vi "未命名 5.vi"() -> ()   [LabVIEW 2012, in "DataGridView.lvlib"]
uses:
  DataGridView.lvlib
panel:
  in  "字符串":string
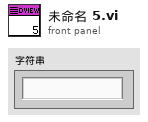
[diagram p1: front panel]
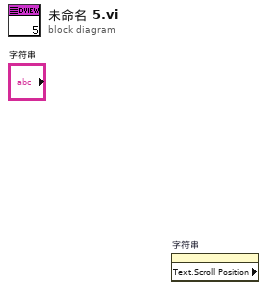
[diagram p0: block diagram]
diagram:
  n1 = property on="字符串" class="Str" props=["Text", "Scroll Position"]() -> ()  [unwired: 2 in, 3 out]
